vi "SetTableHeaderColor.vi"(7 "セル塗?(F)":bool, 8 "エラー入力(エラーなし)":errorcluster, 9 "セル色指定":cluster{"背景色":u32, "文字色":u32}={"背景色"=16448250, "文字色"=0}, 10 "ヘッダー色指定":cluster{"背景色":u32, "文字色":u32}={"背景色"=10210815, "文字色"=0}, 11 "Tbl refnum":refnum<vi>) -> (0 "エラー出力":errorcluster, 3 "Tbl refnum out":refnum<vi>)   [LabVIEW 2014]
uses:
  <vilib>/Utility/miscctls.llb/LVRowAndColumnTypeDef.ctl
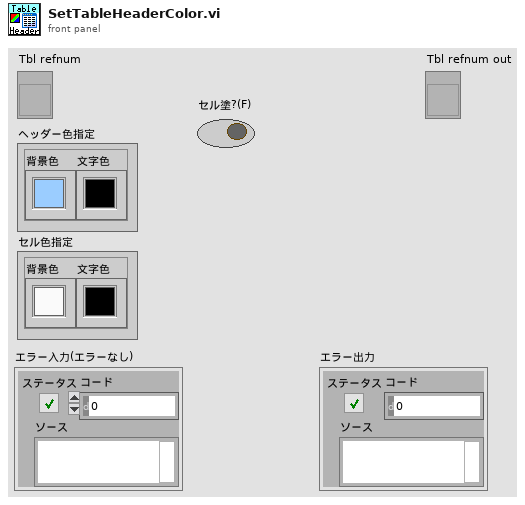
[diagram p1: front panel]
types:
  T1 = typedef "LVRowAndColumnTypeDef.ctl" = cluster{"Row":i32, "Column":i32}
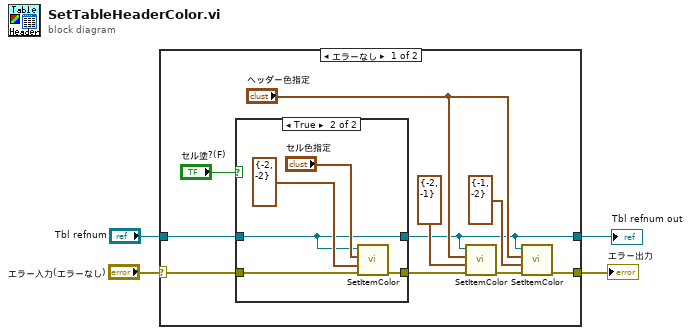
[diagram p0: block diagram]
diagram:
  n1 = case shown="エラーなし" "エラー入力(エラーなし)" {
    selector: "エラー入力(エラーなし)" -> [w9 w23]
    tunnel: [w8 w23] -> w3
    tunnel: "Tbl refnum" -> [w7 w22]
    tunnel: [w5 w22] -> w1
    frame No Error {
      n2 = case shown="TRUE" "セル塗?(F)" {
        tunnel: [w16 w21] -> w10
        tunnel: w9 -> [w16 w18]
        tunnel: w7 -> [w15 w17]
        tunnel: [w15 w17] -> w5
        frame False {
        }
        frame True {
          n3 = call "SetItemColor.vi"("エラー入力(エラーなし)"=w18, "行列指定"=T1 {"Row"=-2, "Column"=-2}, "色指定"="セル色指定", "Tbl refnum"=w17) -> ("エラー出力"=w21:errorcluster)  [unwired: 6 in, 1 out]
        }
      }
      n4 = call "SetItemColor.vi"("エラー入力(エラーなし)"=w10, "行列指定"=T1 {"Row"=-2, "Column"=-1}, "色指定"="ヘッダー色指定", "Tbl refnum"=w5) -> ("エラー出力"=w11:errorcluster)  [unwired: 6 in, 1 out]
      n5 = call "SetItemColor.vi"("エラー入力(エラーなし)"=w11, "行列指定"=T1 {"Row"=-1, "Column"=-2}, "色指定"="ヘッダー色指定", "Tbl refnum"=w5) -> ("エラー出力"=w8:errorcluster)  [unwired: 6 in, 1 out]
    }
    frame Error {
    }
  }
  "エラー出力" <- w3
  "Tbl refnum out" <- w1
